vi "test_Create Instrument Addon from Config with Error.vi"(8 "error in (no error)":errorcluster, 11 "TestCase in":refnum<class "Instrument Addon Scripting API Custom Device Unit Tests.lvclass">) -> (0 "error out":errorcluster, 3 "TestCase out":refnum<class "Instrument Addon Scripting API Custom Device Unit Tests.lvclass">)   [LabVIEW 2019, in "Instrument Addon Scripting API Custom Device Unit Tests.lvclass"]
uses:
  Instrument Addon Scripting API Custom Device Unit Tests.lvclass
  Instrument Addon Scripting API Custom Device Unit Tests.lvclass/Instrument Addon Scripting API Custom Device Unit Tests.ctl
  <vilib>/addons/_JKI Toolkits/VI Tester/TestCase.llb/TestCase.lvclass
  Instrument Addon Scripting API Test Assets/Instrument Addon Scripting API Test Assets.lvclass
  APIs/Scripting API/Instrument Addon Scripting API.lvlib
  C:/Program Files (x86)/National Instruments/LabVIEW 2019/vi.lib/addons/_JKI Toolkits/VI Tester/TestCase.llb/TestCase.lvclass
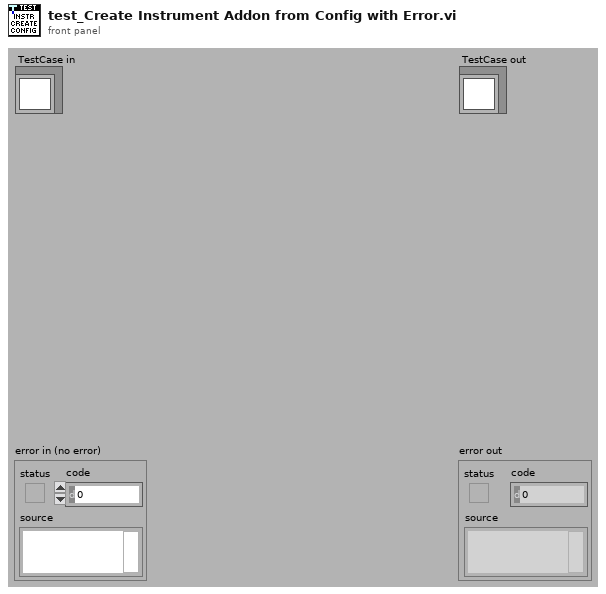
[diagram p1: front panel]
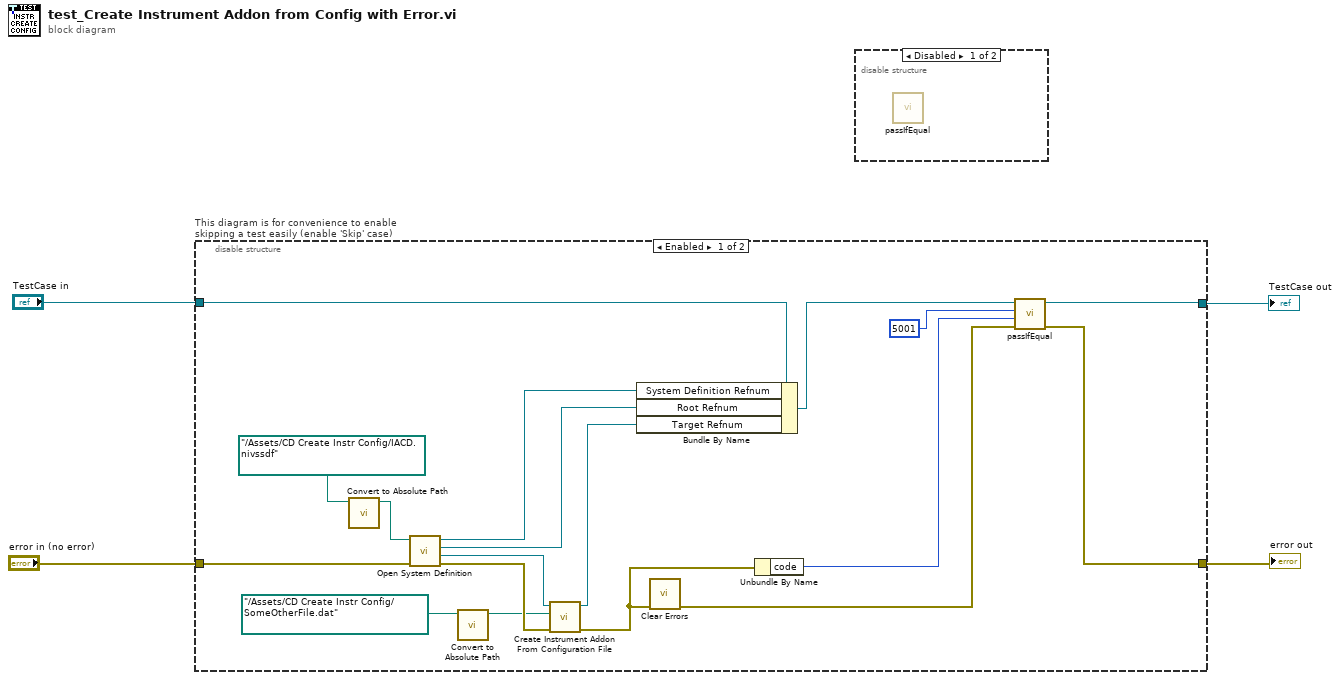
[diagram p0: block diagram]
diagram:
  n1 = disable-structure "This diagram is for convenience to enable skipping a test easily (enable 'Skip' case)" shown="Enabled" {
    disable-tunnel: "TestCase in" -> [w11 w26]
    disable-tunnel: [w13 w24] -> w1
    disable-tunnel: [w12 w25] -> w3
    disable-tunnel: "error in (no error)" -> [w22 w23]
    frame Enabled {
      n2 = call "Convert to Absolute Path.vi"("System Definition File"=path "../Assets/CD Create Instr Config/IACD.nivssdf" ("SDF file")) -> ("Absolute Path"=w20:path)  [unwired: 10 in]
      n3 = call "Open System Definition.vi"("error in (no error)"=w22, "System Definition File"=w20) -> ("error out"=w18:errorcluster, "Target Refnum"=w6:refnum<k24>, "Root Refnum"=w8:refnum<k24>, "System Definition Refnum"=w9:refnum<k24>)  [unwired: 6 in]
      n4 = call "Convert to Absolute Path.vi"("System Definition File"=path "../Assets/CD Create Instr Config/SomeOtherFile.dat" ("SDF file")) -> ("Absolute Path"=w7:path)  [unwired: 10 in]
      n5 = call "Create Instrument Addon From Configuration File.vi"("error in (no error)"=w18, "configuration file path"=w7, "target in"=w6) -> ("error out"=w16:errorcluster, "target out"=w5:refnum<k24>)  [unwired: 6 in, 1 out]
      n6 = Bundle By Name(cluster=w11, "System Definition Refnum"=w9, "Root Refnum"=w8, "Target Refnum"=w5) -> (w10:refnum<class "Instrument Addon Scripting API Custom Device Unit Tests.lvclass">)
      n7 = call <vilib>:"Clear Errors.vi"("error in (no error)"=w16) -> ("error out"=w17:errorcluster)  [unwired: 5 in, 1 out]
      n8 = Unbundle By Name(w16) -> ("code"=w14:i32)
      n9 = call-dynamic "passIfEqual.vi"("error in (no error)"=w17, "y"=w14, "x"=5001 ("code"), "TestCase in"=w10) -> ("error out"=w12:errorcluster, "TestCase out"=w13:refnum<class "Instrument Addon Scripting API Custom Device Unit Tests.lvclass">)  [unwired: 6 in]
    }
    frame Disabled {
      # "skip test result while test is under development"
      n10 = call <vilib>:"skip.vi"("error in (no error)"=w23, "TestCase in"=w26) -> ("error out"=w25:errorcluster, "TestCase out"=w24:refnum<class "Instrument Addon Scripting API Custom Device Unit Tests.lvclass">)  [unwired: 8 in]
    }
  }
  "error out" <- w3
  "TestCase out" <- w1
  n11 = disable-structure shown="Disabled" {
    frame Disabled {
      n12 = call-dynamic "passIfEqual.vi"() -> ()  [unwired: 10 in, 2 out]
    }
    frame Enabled {
    }
  }
